vi "Get Project Hierarchy.vi"(7 "Flat Constructors?":bool, 8 "error in (no error)":errorcluster, 11 "Project Path":path) -> (0 "error out":errorcluster, 1 "Actual Locations":path[](array[path]), 3 "Expected Locations":path[](array[path]))   [LabVIEW 2023]
doc: "Gets the project hierarchy for the LabVIEW project identified by <B>Project Path</B>."
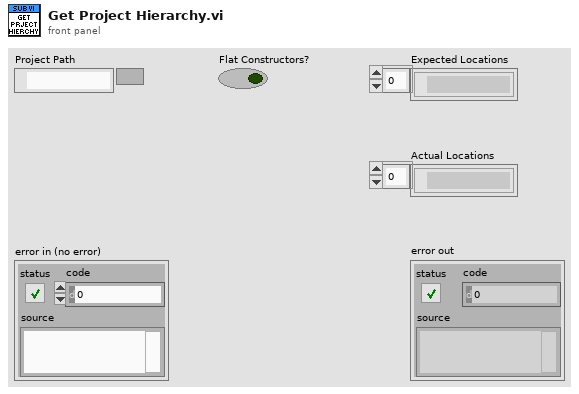
[diagram p1: front panel]
types:
  T1 = typedef "Item Info.ctl" = cluster{"Name":string, "Type":string, "Disk Path":path, "Virtual Path":string}
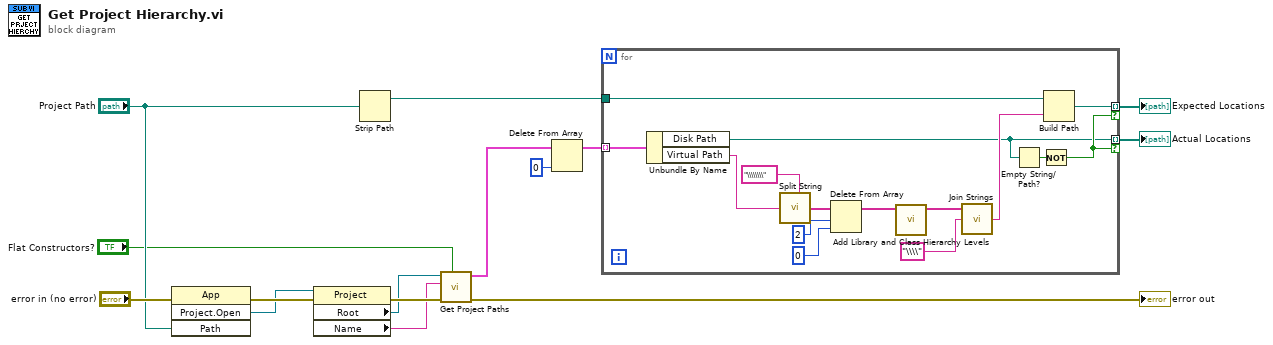
[diagram p0: block diagram]
diagram:
  n1 = invoke class="App" method="Project.Open"(error in="error in (no error)", "Path"="Project Path") -> (error out=w13:errorcluster, "Project:Open"=w11:refnum<vi>)  [unwired: 2 in, 2 out]
  n2 = property class="Project"(reference=w11, error in=w13) -> (error out=w15:errorcluster, "Root"=w10:refnum<vi>, "Name"=w9:string)  [unwired: 1 out]
  n3 = Strip Path(path="Project Path") -> (stripped path=w7:path)  [unwired: 1 out]
  n4 = call "Get Project Paths.vi"("Flat Constructors?"="Flat Constructors?", "error in (no error)"=w15, "Current Virtual Path"=w9, "ProjectItem refnum"=w10) -> ("error out"=→"error out":errorcluster, "Item Info"=w3:T1[])  [unwired: 6 in]
  n5 = Delete From Array(array=w3, index=0) -> (array with subset deleted=w2:T1[])  [unwired: 1 in, 1 out]
  n6 = for {
    tunnel: w2 -> [w18] mode=indexing
    tunnel: [w17] -> w5 mode=indexing if=w20
    tunnel: w7 -> [w25]
    tunnel: [w22] -> w6 mode=indexing if=w20
    n7 = Unbundle By Name(w18) -> ("Disk Path"=w17:path, "Virtual Path"=w16:string)
    n8 = call <vilib>:"Split String.vi"("Split Pattern"="\\\\\\\\", "Input String"=w16) -> ("Split String"=w29:string[])  [unwired: 5 in]
    n9 = Delete From Array(array=w29, length=2 ("index"), index=0) -> (array with subset deleted=w28:string[])  [unwired: 1 out]
    n10 = call "Add Library and Class Hierarchy Levels.vi"("Hierarchy Array"=w28) -> ("Modified Hierarchy Array"=w19:string[])  [unwired: 10 in]
    n11 = call <vilib>:"Join Strings.vi"("Separator (,)"="\\\\" ("Split Pattern"), "Strings In"=w19) -> ("String"=w21:string)  [unwired: 1 in]
    n12 = Empty String/Path?(string/path=w17) -> (empty?=w30:bool)
    n13 = Not(x=w30) -> (.not. x?=w20:bool)
    n14 = Build Path(base path=w25, name or relative path=w21) -> (appended path=w22:path)
  }
  "Expected Locations" <- w6
  "Actual Locations" <- w5
